vi "Unpack Control Mouse Leave.vi"(11 "ControlMouseLeaveMsg":refnum<class "ControlMouseLeaveMsg.lvclass">) -> (2 "Time":u32, 3 "Control Label":string, 5 "Ctl Refnum":refnum<vi>)   [LabVIEW 2020, in "MVA Framework.lvlib" / "ActorEvents.lvlib" / "ControlMouseLeaveMsg.lvclass"]
doc: "<License>\nCopyright © 2017 Composed Systems, LLC | All rights reserved\nwww.composed.io\n\nAuthor: Ethan Stern <ethan.stern@composed.io>\n\nThis software is provided \"AS IS\" WITHOUT WARRANTIES, either express or implied, AND IS FOR EDUCATIONAL PURPOSES ONLY.\n</License>"
uses:
  ControlMouseLeaveMsg.lvclass
  ControlMouseLeaveMsg.lvclass/ControlMouseLeaveMsg.ctl
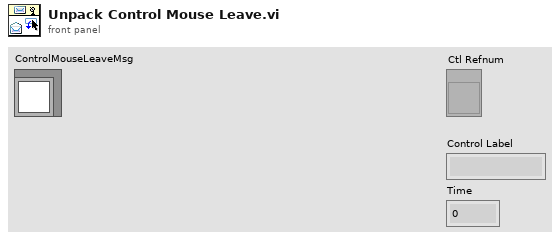
[diagram p1: front panel]
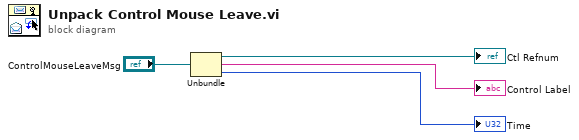
[diagram p0: block diagram]
diagram:
  n1 = Unbundle("ControlMouseLeaveMsg") -> (→"Ctl Refnum":refnum<vi>, →"Control Label":string, →"Time":u32)
